vi "load cache.vi"(8 "error in":errorcluster, 11 "cache path":path) -> (0 "error out":errorcluster, 3 "cache":T1)   [LabVIEW 2013, in "PL_class cache.lvlib"]
uses:
  PL_class cache.lvlib
  cache definition.ctl
  cache search configuration.ctl
  cached class information.ctl
  target class metadata.ctl
  class metadata.ctl
  <vilib>/NI/Tag Bus Module Framework/root configuration/Target Types.ctl
  <vilib>/NI/Tag Bus Module Framework/root configuration/TBM configuration.lvclass
  <vilib>/NI/Configuration Framework/tree serializer/NISE_CEF_TreeSerializer.lvlib
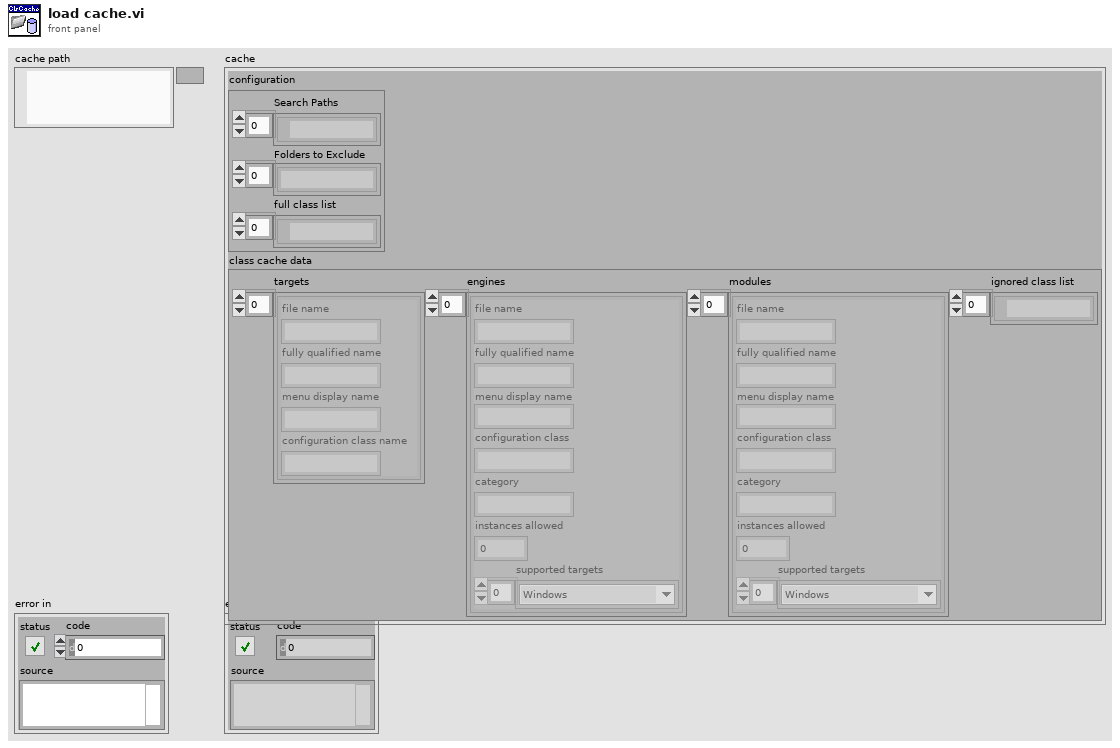
[diagram p1: front panel]
types:
  T1 = typedef "PL_class cache.lvlib/cache definition.ctl" = cluster{"configuration":T2, "class cache data":T3}
  T2 = typedef "PL_class cache.lvlib/cache search configuration.ctl" = cluster{"Search Paths":path[], "Folders to Exclude":string[], "full class list":path[]}
  T3 = typedef "PL_class cache.lvlib/cached class information.ctl" = cluster{"targets":T4[], "engines":T5[], "modules":T5[], "ignored class list":path[]}
  T4 = typedef "PL_class cache.lvlib/target class metadata.ctl" = cluster{"file name":string, "fully qualified name":string, "menu display name":string, "configuration class name":string}
  T5 = typedef "PL_class cache.lvlib/class metadata.ctl" = cluster{"file name":string, "fully qualified name":string, "menu display name":string, "configuration class":string, "category":string, "instances allowed":i32, "supported targets":T6[]}
  T6 = typedef "TBM configuration.lvclass/Target Types.ctl" = enum16{"Windows", "Mac", "Linux", "Linux RT ARM", "VxWorks", "Pharlap", "Other", "Linux RT x64"}
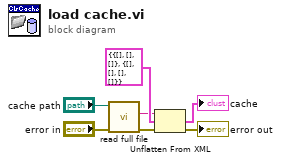
[diagram p0: block diagram]
diagram:
  n1 = call <vilib>:"read full file.vi"("error in"="error in", "file path"="cache path") -> ("error out"=w4:errorcluster, "data"=w3:string)  [unwired: 8 in]
  n2 = Unflatten From XML(xml string=w3, type=T1 {"configuration"={"Search Paths"=[], "Folders to Exclude"=[], "full class list"=[]}, "class cache data"={"targets"=[], "engines"=[], "modules"=[], "ignored class list"=[]}} ("cache"), error in (no error)=w4) -> (value=→"cache":T1, error out=→"error out":errorcluster)
